vi "Choreo_SwerveSample_Equals.vi"(9 "OtherChoreoSwerveSample":T1, 11 "ChoreoSwerveSample":T1) -> (3 "Equal":bool)   [LabVIEW 2019, in "ChoreoLib.lvlib"]
doc: "Determine if two Swerve Trajectory Samples are equal\n\nInputs:\n -- ChoreoSwerveSample - cluster - Swerve sample.\n -- OtherChoreoSwerveSample - cluster - Swerve sample to compare.\n\nOutputs\"\n -- Equal - boolean - TRUE when the samples are the same"
uses:
  ChoreoLib.lvlib
  TypeDef/ChoreoSwerveSample.ctl
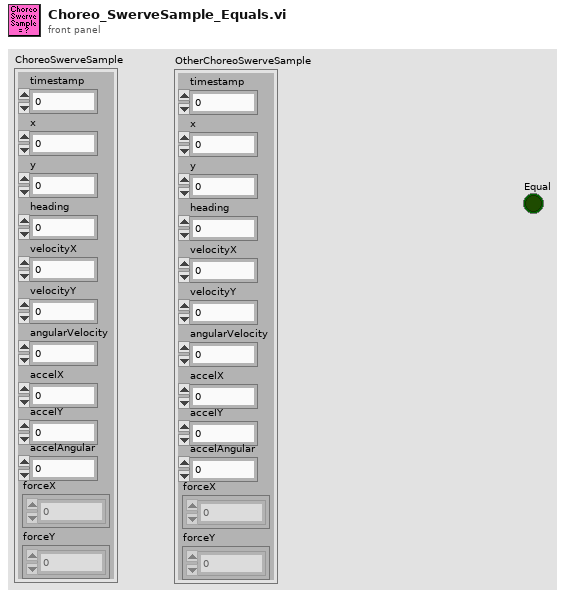
[diagram p1: front panel]
types:
  T1 = typedef "ChoreoLib.lvlib/ChoreoSwerveSample.ctl" = cluster{"timestamp":dbl, "x":dbl, "y":dbl, "heading":dbl, "velocityX":dbl, "velocityY":dbl, "angularVelocity":dbl, "accelX":dbl, "accelY":dbl, "accelAngular":dbl, "forceX":dbl[], "forceY":dbl[]}
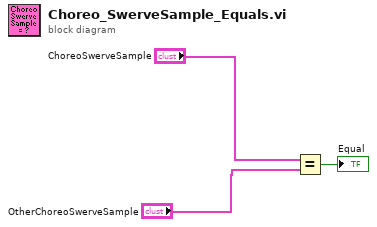
[diagram p0: block diagram]
diagram:
  n1 = Equal?(x="ChoreoSwerveSample", y="OtherChoreoSwerveSample") -> (x = y?=→"Equal":bool)
